vi "Create Events.vi"(11 "Dev Panel in":refnum<class "Dev Panel.lvclass">) -> (0 "error out":errorcluster, 3 "Dev Panel out":refnum<class "Dev Panel.lvclass">)   [LabVIEW 2021, in "Dev Panel.lvclass"]
uses:
  Dev Panel.lvclass
  Dev Panel.lvclass/Dev Panel.ctl
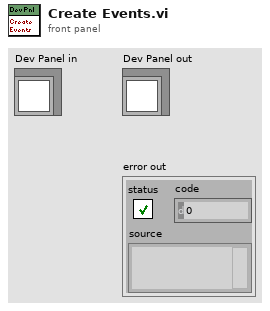
[diagram p1: front panel]
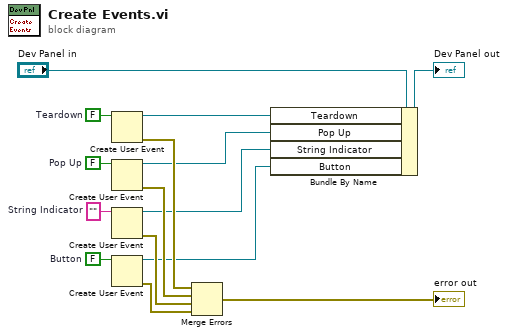
[diagram p0: block diagram]
diagram:
  w10 = FALSE  # Pop Up
  w11 = FALSE  # Button
  w12 = ""  # String Indicator
  w15 = FALSE  # Teardown
  n1 = Create User Event(user event datatype=w15) -> (user event=w14:refnum<user-event>, error out=w13:errorcluster)  [unwired: 1 in]
  n2 = Create User Event(user event datatype=w10) -> (user event=w6:refnum<user-event>, error out=w9:errorcluster)  [unwired: 1 in]
  n3 = Create User Event(user event datatype=w12) -> (user event=w5:refnum<user-event>, error out=w7:errorcluster)  [unwired: 1 in]
  n4 = Create User Event(user event datatype=w11) -> (user event=w4:refnum<user-event>, error out=w8:errorcluster)  [unwired: 1 in]
  n5 = Merge Errors(w13, w9, w7, w8) -> (→"error out":errorcluster)
  n6 = Bundle By Name(cluster="Dev Panel in", "Teardown"=w14, "Pop Up"=w6, "String Indicator"=w5, "Button"=w4) -> (→"Dev Panel out":refnum<class "Dev Panel.lvclass">)
